vi "CHD_TRAJECTORY_DASH_WRITE.vi"   [LabVIEW 2019]
uses:
  CHD_TRAJECTORY_GLOBALS.vi
  <vilib>/Rock Robotics/Network Tables/NT Write Number.vi
  <vilib>/Rock Robotics/Network Tables/NT Write Boolean.vi
  <vilib>/Rock Robotics/Network Tables/NT Write Numeric Array.vi
types:
  T1 = typedef "Trajectory_Library.lvlib/POSE2D.ctl" = cluster{"TRANSLATION":T2, "ROTATION":T3}
  T2 = typedef "Trajectory_Library.lvlib/TRANSLATION2D.ctl" = cluster{"X":dbl, "Y":dbl}
  T3 = typedef "Trajectory_Library.lvlib/ROTATION2D.ctl" = cluster{"VALUE":dbl, "COS":dbl, "SIN":dbl}
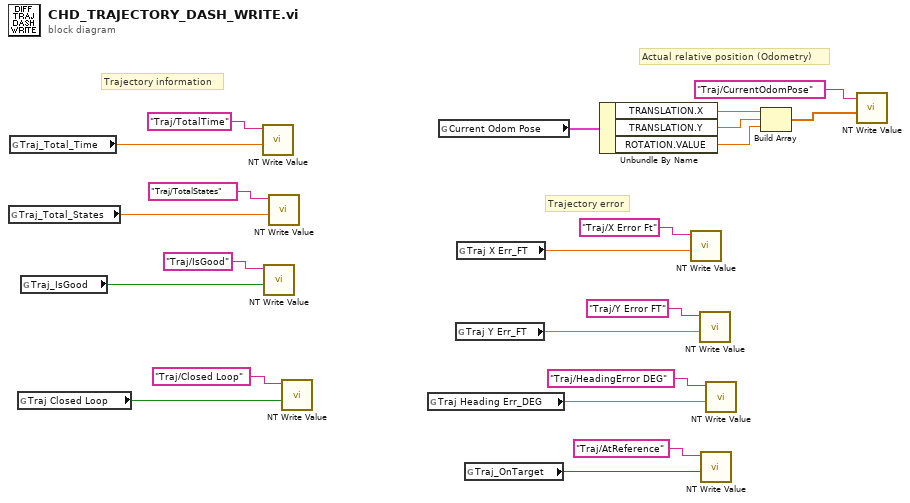
[diagram p0: block diagram]
diagram:
  # "Trajectory information"
  # "Actual relative position (Odometry)"
  # "Trajectory error"
  n1 = global read "CHD_TRAJECTORY_GLOBALS.vi" "Traj_Total_States"() -> (w8:dbl)
  n2 = global read "CHD_TRAJECTORY_GLOBALS.vi" "Traj_Total_Time"() -> (w7:dbl)
  n3 = global read "CHD_TRAJECTORY_GLOBALS.vi" "Traj Closed Loop"() -> (w6:bool)
  n4 = global read "CHD_TRAJECTORY_GLOBALS.vi" "Traj_IsGood"() -> (w9:bool)
  n5 = call-poly <vilib>:"NT Write Value.vi"("value"=w7, "name"="Traj/TotalTime" ("Name")) -> ()  [unwired: 9 in, 1 out]
  n6 = call-poly <vilib>:"NT Write Value.vi"("value"=w9, "name"="Traj/IsGood" ("Name")) -> ()  [unwired: 9 in, 1 out]
  n7 = call-poly <vilib>:"NT Write Value.vi"("value"=w8, "name"="Traj/TotalStates" ("Name")) -> ()  [unwired: 9 in, 1 out]
  n8 = call-poly <vilib>:"NT Write Value.vi"("value"=w6, "name"="Traj/Closed Loop" ("Name")) -> ()  [unwired: 9 in, 1 out]
  n9 = global read "CHD_TRAJECTORY_GLOBALS.vi" "Traj Heading Err_DEG"() -> (w3:dbl)
  n10 = global read "CHD_TRAJECTORY_GLOBALS.vi" "Current Odom Pose"() -> (w1:T1)
  n11 = global read "CHD_TRAJECTORY_GLOBALS.vi" "Traj Y Err_FT"() -> (w5:dbl)
  n12 = global read "CHD_TRAJECTORY_GLOBALS.vi" "Traj X Err_FT"() -> (w4:dbl)
  n13 = global read "CHD_TRAJECTORY_GLOBALS.vi" "Traj_OnTarget"() -> (w2:bool)
  n14 = Unbundle By Name(w1) -> ("TRANSLATION.X"=w19:dbl, "TRANSLATION.Y"=w20:dbl, "ROTATION.VALUE"=w21:dbl)
  n15 = call-poly <vilib>:"NT Write Value.vi"("value"=w4, "name"="Traj/X Error Ft" ("Name")) -> ()  [unwired: 9 in, 1 out]
  n16 = call-poly <vilib>:"NT Write Value.vi"("value"=w5, "name"="Traj/Y Error FT" ("Name")) -> ()  [unwired: 9 in, 1 out]
  n17 = call-poly <vilib>:"NT Write Value.vi"("value"=w2, "name"="Traj/AtReference" ("Name")) -> ()  [unwired: 9 in, 1 out]
  n18 = call-poly <vilib>:"NT Write Value.vi"("value"=w3, "name"="Traj/HeadingError DEG" ("Name")) -> ()  [unwired: 9 in, 1 out]
  n19 = Build Array(w19, w20, w21) -> (w17:dbl[])
  n20 = call-poly <vilib>:"NT Write Value.vi"("value"=w17, "name"="Traj/CurrentOdomPose" ("Name")) -> ()  [unwired: 9 in, 1 out]
